vi "Configure Math Scaling.vi"(5 "Auto Tracking (T: Enable)":bool=TRUE, 6 "Range (1E-6)":dbl=1e-06, 7 "Horizontal/Vertical (0: Horizontal)":u16(ring) items=["Horizontal", "Vertical"], 8 "error in (no error)":errorcluster, 9 "Position/Offset (0.0 )":dbl, 10 "Math Channel (0: Function 1)":i32(ring) items=["Function 1", "Function 2", "Function 3", "Function 4", "Function 5", "Function 6", "Function 7", "Function 8", "Function 9", "Function 10", "Function 11", "Function 12", "Function 13", "Function 14", "Function 15", "Function 16"], 11 "VISA resource name":refnum<visa-resource-name>) -> (0 "error out":errorcluster, 3 "VISA resource name out":refnum<visa-resource-name>)   [LabVIEW 2020, in "Agilent 90000 Series.lvlib"]
doc: "Configures horizontal and vertical characteristics for math operation."
uses:
  Agilent 90000 Series.lvlib
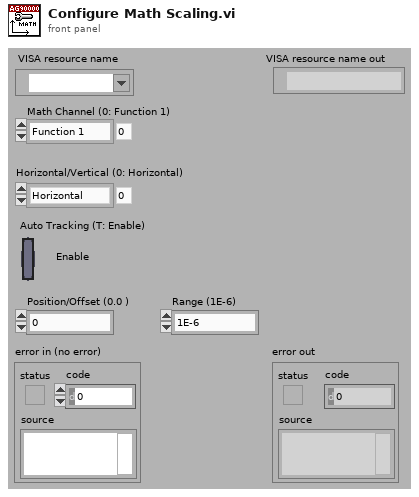
[diagram p1: front panel]
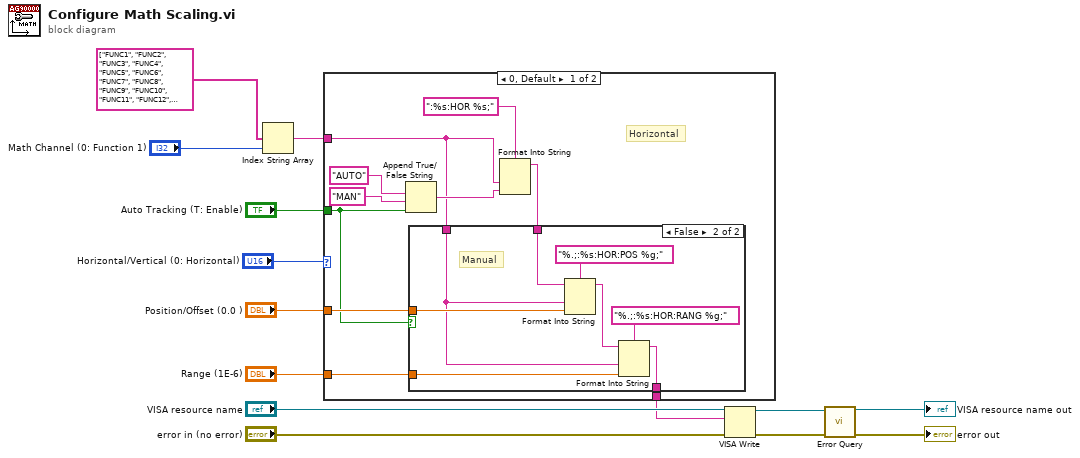
[diagram p0: block diagram]
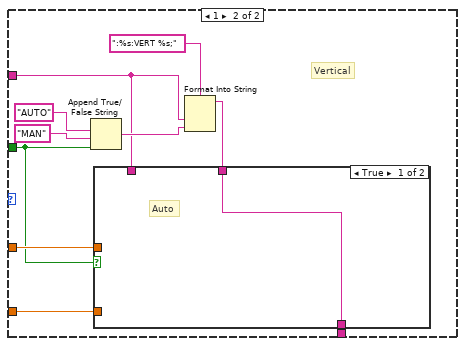
[diagram p3: hidden frame]
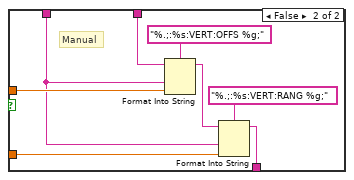
[diagram p4: hidden frame]
diagram:
  n1 = Index String Array(1:"Math Channel (0: Function 1)", 2:string[] ["FUNC1", "FUNC2", "FUNC3", "FUNC4", "FUNC5", "FUNC6", "FUNC7", "FUNC8", "FUNC9", "FUNC10", "FUNC11", "FUNC12", "FUNC13", "FUNC14", "FUNC15", "FUNC16"] ("subarray 2")) -> (0:w6:string)  [unwired: 1 in]
  n2 = case shown="0, Default" "Horizontal/Vertical (0: Horizontal)" {
    tunnel: "Position/Offset (0.0 )" -> [w20 w39]
    tunnel: w6 -> [w19 w38]
    tunnel: "Range (1E-6)" -> [w18 w37]
    tunnel: [w16 w35] -> w4
    tunnel: "Auto Tracking (T: Enable)" -> [w15 w34]
    frame 0, Default {
      # "Horizontal"
      n3 = Append True/False String(1:w15, 2:"MAN" ("false string"), 3:"AUTO" ("true string")) -> (0:w21:string)  [unwired: 1 out]
      n4 = Format Into String(format string=":%s:HOR %s;", w19, w21) -> (resulting string=w17:string)  [unwired: 2 in, 1 out]
      n5 = case shown="False" w15 {
        tunnel: w20 -> [_ w32]
        tunnel: w19 -> [_ w30]
        tunnel: w18 -> [_ w29]
        tunnel: w17 -> [w25 w27]
        tunnel: [w25 w26] -> w16
        frame True {
          # "Auto"
        }
        frame False {
          # "Manual"
          n6 = Format Into String(format string="%.;:%s:HOR:POS %g;", initial string=w27, w30, w32) -> (resulting string=w28:string)  [unwired: 1 in, 1 out]
          n7 = Format Into String(format string="%.;:%s:HOR:RANG %g;", initial string=w28, w30, w29) -> (resulting string=w26:string)  [unwired: 1 in, 1 out]
        }
      }
    }
    frame 1 {
      # "Vertical"
      n8 = Append True/False String(1:w34, 2:"MAN" ("false string"), 3:"AUTO" ("true string")) -> (0:w40:string)  [unwired: 1 out]
      n9 = Format Into String(format string=":%s:VERT %s;", w38, w40) -> (resulting string=w36:string)  [unwired: 2 in, 1 out]
      n10 = case shown="True" w34 {
        tunnel: w39 -> [_ w51]
        tunnel: w38 -> [_ w49]
        tunnel: w37 -> [_ w48]
        tunnel: w36 -> [w44 w46]
        tunnel: [w44 w45] -> w35
        frame True {
          # "Auto"
        }
        frame False {
          # "Manual"
          n11 = Format Into String(format string="%.;:%s:VERT:OFFS %g;", initial string=w46, w49, w51) -> (resulting string=w47:string)  [unwired: 1 in, 1 out]
          n12 = Format Into String(format string="%.;:%s:VERT:RANG %g;", initial string=w47, w49, w48) -> (resulting string=w45:string)  [unwired: 1 in, 1 out]
        }
      }
    }
  }
  n13 = VISA Write(VISA resource name="VISA resource name", write buffer=w4, error in (no error)="error in (no error)") -> (VISA resource name out=w12:refnum<visa-resource-name>, error out=w11:errorcluster)  [unwired: 1 out]
  n14 = call "Error Query.vi"("error in (no error)"=w11, "VISA resource name"=w12) -> ("error out"=→"error out":errorcluster, "VISA resource name out"=→"VISA resource name out":refnum<visa-resource-name>)  [unwired: 8 out]
